vi "Dashboard Main.vi"() -> ()   [LabVIEW 2014]
uses:
  Camera Types.ctl
  <vilib>/event_ctls.llb/eventvkey.ctl
  <vilib>/Rock Robotics/WPI/Dashboard/WPI_DashboardLogging Global.vi
  <vilib>/Rock Robotics/Network Tables/SD Write Number.vi
  <vilib>/Rock Robotics/Network Tables/SD Read Number.vi
  <vilib>/Rock Robotics/Network Tables/SD Write Boolean.vi
  <vilib>/Rock Robotics/Network Tables/SD Read String.vi
  <vilib>/Rock Robotics/Network Tables/SD Write String.vi
  <vilib>/Utility/config.llb/Write Key (String).vi
  <vilib>/Utility/config.llb/Write Key (I32).vi
  <vilib>/Utility/config.llb/NI_LVConfig.lvlib
  <vilib>/vision/NI_Vision_Development_Module.lvlib
panel:
  in  "Limit Tests?":bool
  in  "Camera Type":T1=enum."MS HD3000 square"
  in  "Aspect Fudge Factor":dbl=1.0
  in  "Score Threshold":dbl=75.0
  in  "Show Carpet Mask":bool
  in  "Carpet Color":T2(tab)
  in  "Red":T3={"Hue"={231.0, 14.0}, "Sat"={83.0, 255.0}, "Val"={52.5, 255.0}} {"Hue" scale=0.0..255.0 scale format="%#_3g"}
  in  "Blue":T3={"Hue"={119.0, 181.0}, "Sat"={33.0, 255.0}, "Val"={48.571428571428584, 255.0}} {"Hue" scale=0.0..255.0 scale format="%#_3g"}
  out "Sorted Scores":T4(array[cluster]) {"Carpet" format="%#_3g"; "S" format="%#_3g"; "Trapezoid %" format="%#_3g"; "L" format="%#_3g"; "Area to CH" format="%#_3g"; "X" format="%#_3g"; "Y" format="%#_3g"}
  out "Particles":i32
  out "Masked":T5(plugin-control)
  in  "TCP":refnum<k5>
  in  "Rec Mode":enum32{"Stop", "Record", "Playback"}(radio)
  in  "Vision":u16(ring) items=["Camera Off", "USB Camera SW", "USB Camera HW", "IP Camera"]
  out "Camera IP":string
  out "Image Message":string="Timeout in Camera Communications"
  in  "Dashboard Tab":T6(tab)
  in  "AutonTotePush":bool
  in  "Encoder Reset":bool
  in  "Gyro Reset":bool
  in  "Auton Select":string(combo)="Blank 1"
  out "Drive Mode":string
  in  "Is Logitech":bool
  out "Lift Height":dbl(slide) scale=0.0..4.0
  in  "Camera Settings":T7={"Frame Rate"=30, "Compression"=30, "Size"=1} {"Frame Rate" scale=1.0..30.0; "Size" items=["640x480", "320x240", "160x120"]}
  out "MotorChart R":cluster{"Numeric":dbl, "Numeric":dbl}(graph)
  out "MotorChart L":T8(graph)
  out "MotorSliders R":cluster{"MotorSlide1":dbl, "MotorSlide2":dbl} {"MotorSlide2" scale=-1.0..1.0 scale format="%#_2e"; "MotorSlide1" scale=-1.0..1.0 scale format="%#_2e"}
  out "MotorSliders L":T9 {"MotorSlide4 2" scale=0.0..14.0 scale format="%#_2e"; "MotorSlide2" scale=-1.0..1.0 scale format="%#_2e"; "MotorSlide1" scale=-1.0..1.0 scale format="%#_2e"}
  out "Gyro":dbl(knob) scale=0.0..360.0
  out "JS1 Z":dbl(slide) scale=-1.0..1.0 scale format="%#_2e"
  out "JS1 Graph":cluster{"X":dbl, "Y":dbl}[](graph)
  out "JS1 Buttons":T10
  out "JS2 Z":dbl(slide) scale=-1.0..1.0 scale format="%#_2e"
  out "JS2 Graph":cluster{"X":dbl, "Y":dbl}[](graph)
  out "JS2 Buttons":T10
  out "Mode":T11(ring)=enum."Auto Disabled"
  in  "DB Camera Config":bool
  out "fps":dbl format="%#.1g"
  out "Mbps":dbl format="%#.1g"
  out "Mbps 2":bool
  in  "DB/String 9":string
  in  "DB/String 8":string
  in  "DB/String 7":string
  in  "DB/String 6":string
  in  "DB/String 5":string
  in  "DB/String 4":string
  in  "DB/String 3":string
  in  "DB/String 2":string
  in  "DB/String 1":string
  in  "DB/String 0":string
  in  "DB/Slider 0":dbl(slide) scale=0.0..5.0
  in  "DB/Slider 1":dbl(slide) scale=0.0..5.0
  in  "DB/Slider 2":dbl(slide) scale=0.0..5.0
  in  "DB/Slider 3":dbl(slide) scale=0.0..5.0
  out "DB/LED 3":bool
  out "DB/LED 2":bool
  out "DB/LED 1":bool
  out "DB/LED 0":bool
  in  "DB/Button 3":bool
  in  "DB/Button 2":bool
  in  "DB/Button 1":bool
  in  "DB/Button 0":bool caption="New Name"
  out "Amp Chart":dbl(graph)
  in  "Lift override":bool
  out "Left Lift Current":dbl
  out "Right Lift Current":dbl
  in  "Test Slider":dbl(slide) scale=0.0..100.0 scale format="%#_3g"
  in  "On/Off":bool caption="Solenoid"
  in  "Test Name":u16(ring) items=["Select the test to run...", "Example Test", "-------------------------------", "List of tests is built in robot code.", "Replace with your own automated tests."]
  in  "Test Tree":string(tree)
  in  "Motor":cluster{"Value":dbl, "Enable":bool} {"Value" scale=-1.0..1.0 scale format="%#_3g"}
  out "Progress":T12 {"Test Progress" scale=0.0..100.0}
  in  "Rev/Fwd":cluster{"Forward":bool, "Reverse":bool}
  in  "Test Ring":u16(ring) items=["Monochrome", "Color"]
  in  "Listbox":i32(listbox)
  out "Tree":string(tree)
  in  "Tote Color":T3={"Hue"={23.67058792990901, 48.923317529462665}, "Sat"={66.78571428571429, 255.0}, "Val"={48.571428571428584, 255.0}} {"Hue" scale=0.0..255.0 scale format="%#_3g"}
  in  "Annotate":bool
  out "Detected Totes":T13(array[cluster]) {"Normalized Rect"."Numeric 5" format="%#_2g"; "Normalized Rect"."Numeric 3" format="%#_2g"; "Normalized Rect"."Numeric 2" format="%#_2g"; "Normalized Rect"."Numeric" format="%#_2g"}
  out "Camera Image":T5(plugin-control)
  out "Boolean":bool
  # "Aspect Ratio"
  # "Density Profile"
  # "Left"
  # "Front"
  # "Right"
  # "Battery"
  # "This tab is a great place for autonomous settings and robot-specific values.\nPlace controls and indicators inside this tab and match name to\nDashboard Variables on robot. You can also delete this comment."
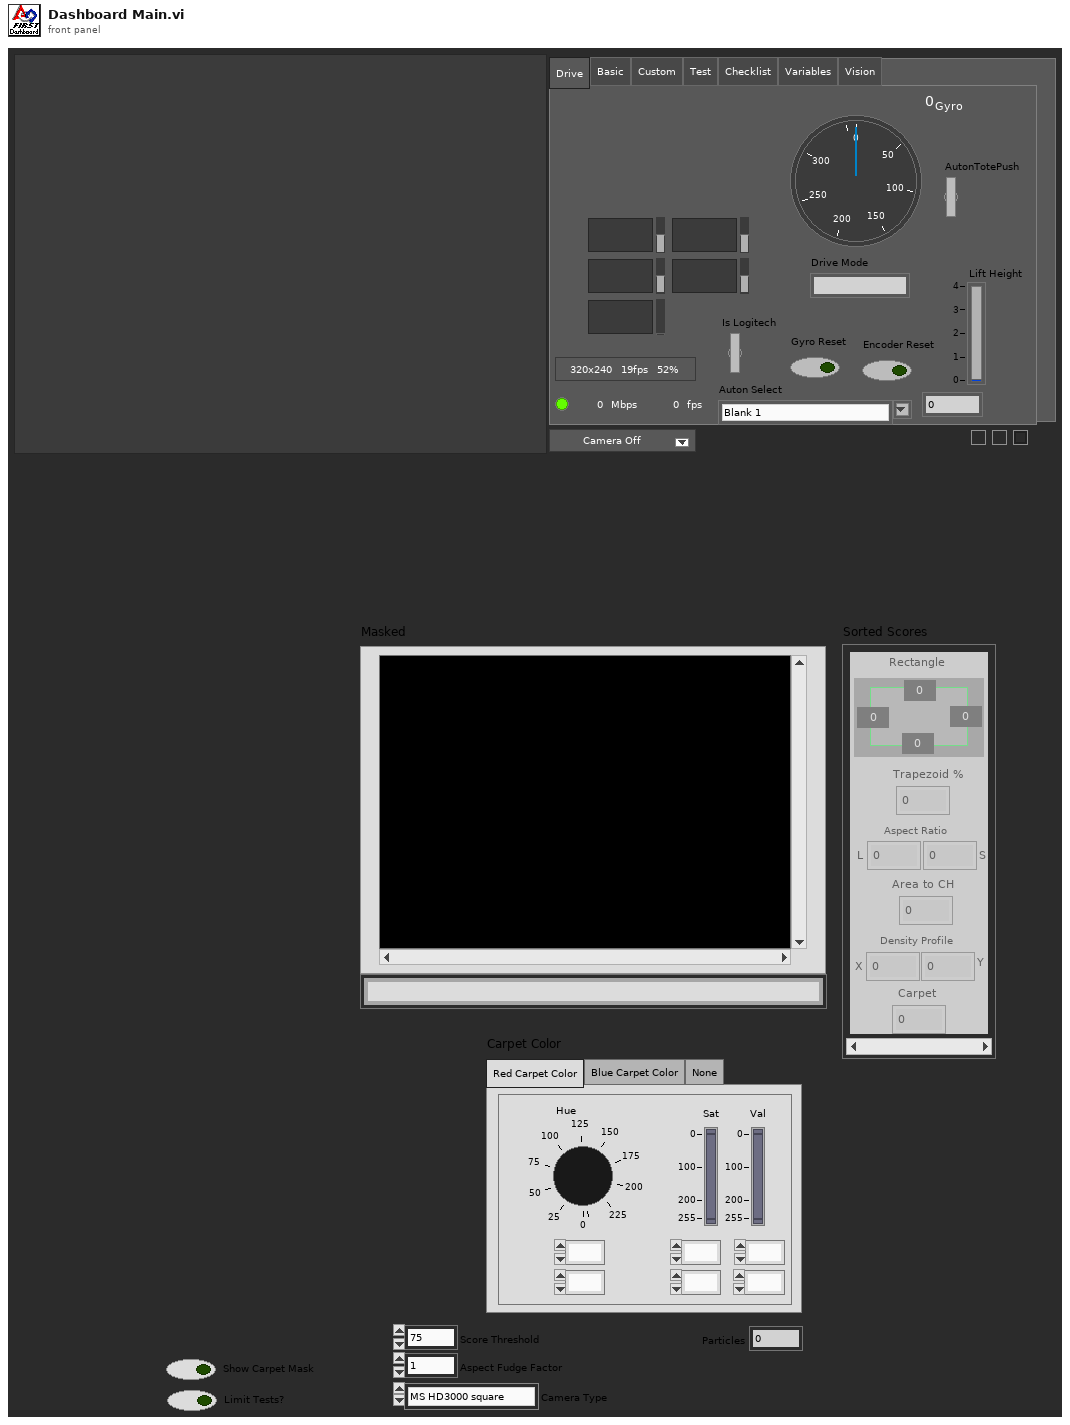
[diagram p1: front panel]
types:
  T1 = typedef "Camera Types.ctl" = enum16{"206", "1011", "1013", "MS HD3000 square", "MS HD3000 640x480"}
  T2 = enum32{"Red Carpet Color", "Blue Carpet Color", "None"}
  T3 = cluster{"Hue":cluster{dbl, dbl}, "Sat":cluster{dbl, dbl}, "Val":cluster{dbl, dbl}}
  T4 = cluster{"Rectangle":cluster{"Numeric":dbl, "Numeric 2":dbl, "Numeric 3":dbl, "Numeric 5":dbl}, "Trapezoid %":dbl, "L":dbl, "S":dbl, "Area to CH":dbl, "X":dbl, "Y":dbl, "Carpet":dbl}[]
  T5 = typedef "IMAQ Image.ctl" = refnum<image>
  T6 = enum32{"Drive", "Basic", "Custom", "Test", "Checklist", "Variables", "Vision"}
  T7 = cluster{"Frame Rate":i32, "Compression":i32, "Size":u16}
  T8 = cluster{"Numeric":dbl, "Numeric":dbl, "Battery V":dbl}
  T9 = cluster{"MotorSlide1":dbl, "MotorSlide2":dbl, "MotorSlide4 2":dbl}
  T10 = cluster{bool, bool, bool, bool, bool, bool, bool, bool, bool, bool, bool, bool}
  T11 = enum8{"Tele-Op Disabled", "Tele-Op Enabled", "Auto Disabled", "Auto Enabled", "Test Disabled", "Test Enabled", "Disconnected", "No Code", "E-Stop"}
  T12 = cluster{"Test Progress":u8, "Test Progress Text":string}
  T13 = cluster{"Distance (ft)":dbl, "Center":cluster{dbl, dbl}, "Normalized Rect":cluster{"Numeric":dbl, "Numeric 2":dbl, "Numeric 3":dbl, "Numeric 5":dbl}}[]
  T14 = typedef "Particle Parameters" = i32
  T15 = typedef "Image Type" = u32
  T16 = enum32{"Drive", "Basic", "Custom", "Test", "Checklist", "Variables"}
  T17 = cluster{"Camera Image":refnum<vi>, "Dashboard Tab":refnum<vi>, "Boolean":refnum<vi>, "Vision":refnum<vi>, "Rec Mode":refnum<vi>, "Test Slider":refnum<vi>, "On/Off ":refnum<vi>, "Test Ring":refnum<vi>, "Rev/Fwd":refnum<vi>, "Test Name":refnum<vi>, "Motor":refnum<vi>, "Progress":refnum<vi>, "CheckList":refnum<vi>, "Tree":refnum<vi>, "Test Tree":refnum<vi>}
  T18 = cluster{"Error Strings":string, "Disable Counts":cluster{u16, u16}, "Rail Faults":cluster{u16, u16, u16}, "Robot IP":string, "DB Mode":u8, "Event Info":cluster{"Name":string, "Type":u8, "Number":u16, "Replay":u8}, "Camera Addr":string}
  T19 = cluster{"Storage":cluster{"Disk Free":u64, "RAM Block":u32, "RAM free":u32}, "CPU Utilization":cluster{"CPU % ISR":sgl, "CPU % Time Crit":sgl, "CPU % Timed Str":sgl, "CPU % High":sgl, "CPU % Above":sgl, "CPU % Normal":sgl, "CPU % Low":sgl}, "CAN":cluster{"% Bus Utilization":sgl, "Bus Off Cnt":u32, "TX_FIFO Full Cnt":u32, "Receive Error Cnt":u8, "Transmit Error Cnt":u8}, "HID":cluster{"HID Outputs":u32, "Rumble Low":u16, "Rumble High":u16}[]}
  T20 = cluster{"Status bits":cluster{"Test Mode":bool, "Autonomous":bool, "Enabled":bool, "Code Start":bool, "Brownout":bool, "Reserved 2":bool, "Reserved 3":bool, "E-Stop":bool}, "Code Trace":cluster{"Disabled":bool, "TeleOp":bool, "Auto":bool, "Test":bool}, "Controller Type":enum16{"unknown", "cRIO", "roboRio"}, "Code?":enum16{"unknown", "noCode", "code"}, "Battery V":dbl}
  T21 = cluster{"Control Bits":cluster{"TestMode":bool, "Autonomous":bool, "Enabled":bool, "FMS Present":bool, bool, bool, bool, "E-Stop":bool}, "Team Station ":u8, "Countdown":sgl, "Joystick Values":cluster{"Axes":dbl[], "Buttons":bool[], "POVs":i16[]}[]}
  T22 = cluster{"Axes":dbl[], "Buttons":bool[], "POVs":i16[]}[]
  T23 = cluster{"Axes":dbl[], "Buttons":bool[], "POVs":i16[]}
  T24 = cluster{"Buttons[0]":bool, "Buttons[1]":bool, "Buttons[2]":bool, "Buttons[3]":bool, "Buttons[4]":bool, "Buttons[5]":bool, "Buttons[6]":bool, "Buttons[7]":bool, "Buttons[8]":bool, "Buttons[9]":bool, "Buttons[10]":bool, "Buttons[11]":bool}
  T25 = cluster{"Bounding box":cluster{"left":dbl, "top":dbl, "right":dbl, "bottom":dbl}, "Trapezoid":dbl, "Long Aspect":dbl, "Short Aspect":dbl, "Area to CH":dbl, "X Mask":dbl, "Y Mask":dbl, "Carpet":dbl}[]
  T26 = cluster{"Red":cluster{"Hue":cluster{dbl, dbl}, "Sat":cluster{dbl, dbl}, "Val":cluster{dbl, dbl}}, "Blue":cluster{"Hue":cluster{dbl, dbl}, "Sat":cluster{dbl, dbl}, "Val":cluster{dbl, dbl}}}
  T27 = cluster{cluster{"[0]":dbl, "[1]":dbl, "[2]":dbl, "[3]":dbl}, "Score":dbl, "Long Edge Score":dbl, "Short Edge Score":dbl, dbl, "X Score":dbl, "Y Score":dbl, "Carpet":dbl}[]
  T28 = cluster{"Distance (ft)":dbl, "Center":cluster{"X":dbl, "Y":dbl}, "Normalized Rect":cluster{"Numeric":dbl, "Numeric 2":dbl, "Numeric 3":dbl, "Numeric 5":dbl}}[]
  T29 = cluster{"Distance (ft)":dbl, "Center":cluster{"X":dbl, "Y":dbl}, "Normalized Rect":cluster{"Numeric":dbl, "Numeric 2":dbl, "Numeric 3":dbl, "Numeric 5":dbl}}
  T30 = typedef "NI_LVConfig.lvlib/Config Data RefNum.ctl" = refnum<k1>
  T31 = cluster{"Operation":enum16{"Update", "Clear"}, "Color Box":u32}[]
  T32 = typedef "eventvkey.ctl" = enum16{"ASCII", "Enter", "Return", "Shift", "Ctrl", "Alt", "Cmd", "Opt", "Caps", "NumLock", "Clear", "Break", "Up", "Down", "Left", "Right", "Insert", "Delete", "Home", "End", "PageUp", "PageDown", "Escape", "Help", "Pause", "ScrollLock", "F1", "F2", "F3", "F4", "F5", "F6", "F7", "F8", "F9", "F10", "F11", "F12", "F13", "F14", "F15", "F16", "F17", "F18", "F19", "F20", "F21", "F22", "F23", "F24", "Play", "VolumeUp", "VolumeDown", "Mute", "Two Byte Char"}
  T33 = cluster{"Image Size":bool, "Image Type":bool, "Pixel Value":bool, "ROI Information":bool, "Zoom Factor":bool}
  T34 = enum8{"Enabled", "Disabled", "Disabled and Grayed Out"}
  T35 = cluster{"Operation":enum16{"Update", "Clear"}, "Color Box":u32}
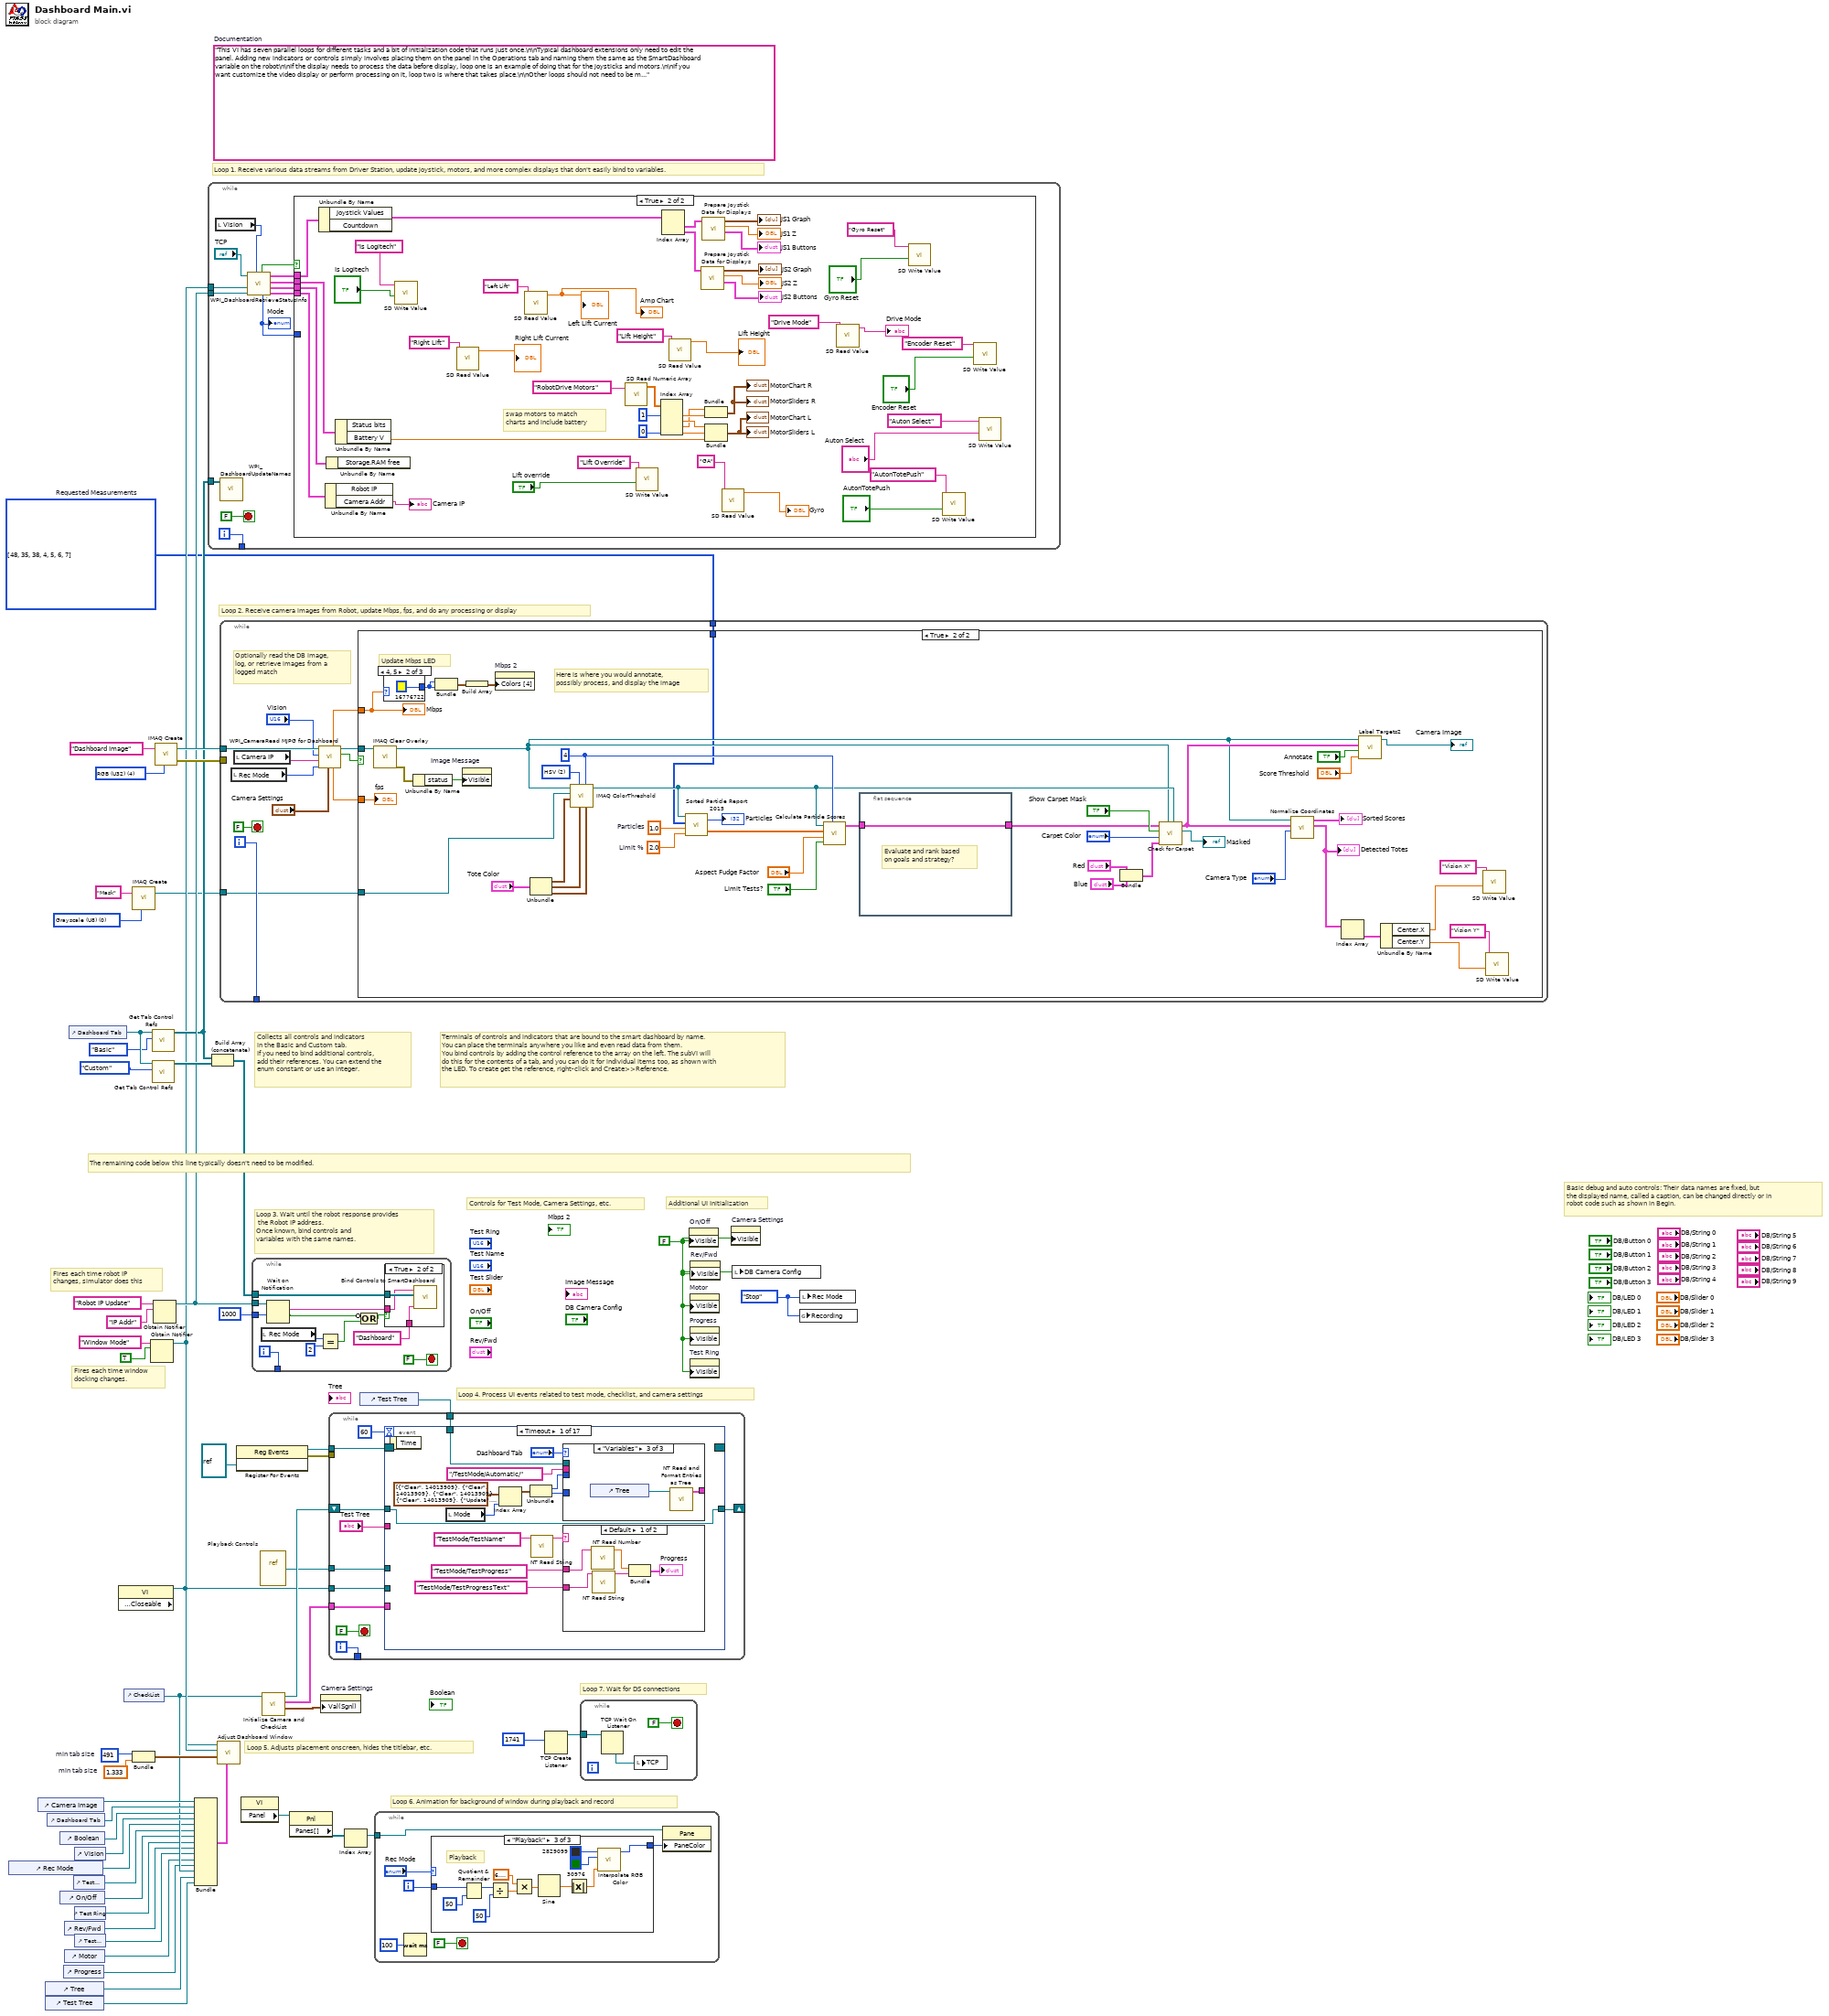
[diagram p0: block diagram]
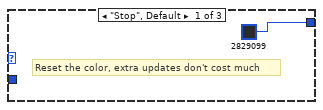
[diagram p3: hidden frame]
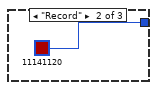
[diagram p4: hidden frame]
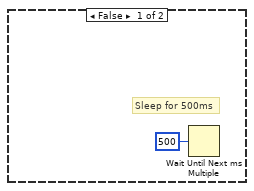
[diagram p6: hidden frame]
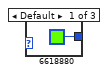
[diagram p7: hidden frame]
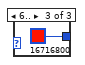
[diagram p8: hidden frame]
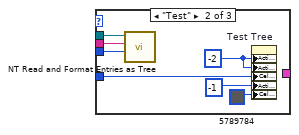
[diagram p10: hidden frame]
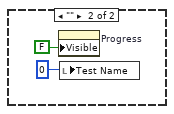
[diagram p11: hidden frame]
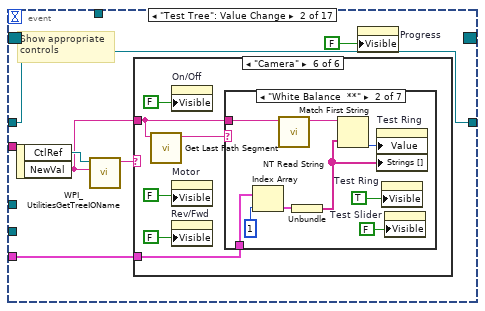
[diagram p12: hidden frame]
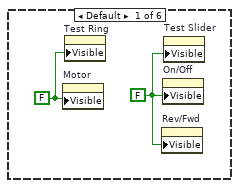
[diagram p13: hidden frame]
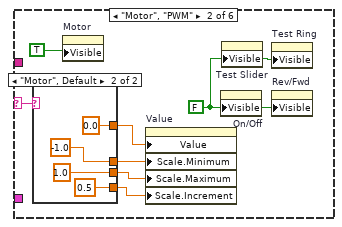
[diagram p14: hidden frame]
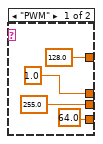
[diagram p15: hidden frame]
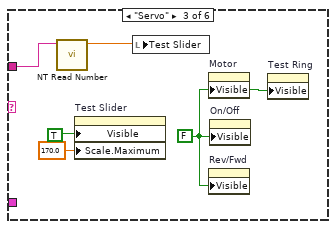
[diagram p16: hidden frame]
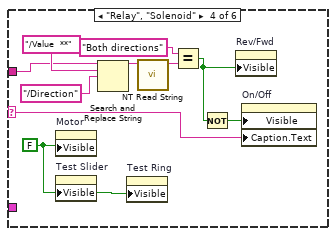
[diagram p17: hidden frame]
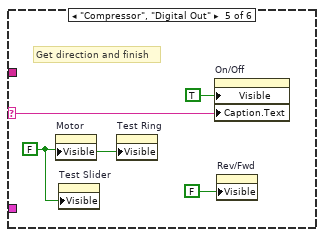
[diagram p18: hidden frame]
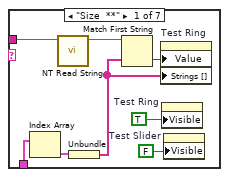
[diagram p19: hidden frame]
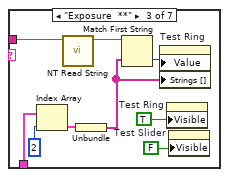
[diagram p20: hidden frame]
diagram:
  w1 = T14[] [48, 35, 38, 4, 5, 6, 7] items=["Center of Mass X", "Center of Mass Y", "First Pixel X", "First Pixel Y", "Bounding Rect Left", "Bounding Rect Top", "Bounding Rect Right", "Bounding Rect Bottom", "Max Feret Diameter Start X", "Max Feret Diameter Start Y", "Max Feret Diameter End X", "Max Feret Diameter End Y", "Max Horiz. Segment Length Left", "Max Horiz. Segment Length Right", "Max Horiz. Segment Length Row", "-", "Bounding Rect Width", "Bounding Rect Height", "Bounding Rect Diagonal", "Perimeter", "Convex Hull Perimeter", "Holes' Perimeter", "Max Feret Diameter", "Equivalent Ellipse Major Axis", "Equivalent Ellipse Minor Axis", "Equivalent Ellipse Minor Axis (Feret)", "Equivalent Rect Long Side", "Equivalent Rect Short Side", "Equivalent Rect Diagonal", "Equivalent Rect Short Side (Feret)", "Average Horiz. Segment Length", "Average Vert. Segment Length", "Hydraulic Radius", "Waddel Disk Diameter", "-", "Area", "Holes' Area", "Particle & Holes' Area", "Convex Hull Area", "Image Area", "-", "Number of Holes", "Number of Horiz. Segments", "Number of Vert. Segments", "-", "Orientation", "Max Feret Diameter Orientation", "-", "% Area/Image Area", "% Area/(Particle & Holes' Area)", "Ratio of Equivalent Ellipse Axes", "Ratio of Equivalent Rect Sides", "-", "Elongation Factor", "Compactness Factor", "Heywood Circularity Factor", "Type Factor", "-", "Sum X", "Sum Y", "Sum XX", "Sum XY", "Sum YY", "Sum XXX", "Sum XXY", "Sum XYY", "Sum YYY", "-", "Moment of Inertia XX", "Moment of Inertia XY", "Moment of Inertia YY", "Moment of Inertia XXX", "Moment of Inertia XXY", "Moment of Inertia XYY", "Moment of Inertia YYY", "Norm. Moment of Inertia XX", "Norm. Moment of Inertia XY", "Norm. Moment of Inertia YY", "Norm. Moment of Inertia XXX", "Norm. Moment of Inertia XXY", "Norm. Moment of Inertia XYY", "Norm. Moment of Inertia YYY", "Hu Moment 1", "Hu Moment 2", "Hu Moment 3", "Hu Moment 4", "Hu Moment 5", "Hu Moment 6", "Hu Moment 7"]  # Requested Measurements
  w4 = T15 0 items=["Grayscale (U8)", "Grayscale (I16)", "Grayscale (SGL)", "Complex (CSG)", "RGB (U32)", "HSL (U32)", "RGB (U64)", "Grayscale (U16)"] ("Image Type")
  w28 = 491  # min tab size
  w27 = 1.333  # min tab size
  w36 = enum32{"Stop", "Record", "Playback"}."Stop" ("Rec Mode")
  w10 = FALSE ("Visible")
  (unwired) "This VI has seven parallel loops for different tasks and a bit of initialization code that runs just once.\n\nTypical dashboard extensions only need to edit the panel. Adding new indicators or controls simply involves placing them on the panel in the Operations tab and naming them the same as the SmartDashboard variable on the robot\n\nIf the display needs to process the data before display, loop one is an example of doing that for the joysticks and motors.\n\nIf you want customize the video display or perform processing on it, loop two is where that takes place.\n\nOther loops should not need to be modified. They are pretty standard, and document the task they perform."  # Documentation
  w56 = T15 4 items=["Grayscale (U8)", "Grayscale (I16)", "Grayscale (SGL)", "Complex (CSG)", "RGB (U32)", "HSL (U32)", "RGB (U64)"] ("Image Type")
  # "Loop 7. Wait for DS connections"
  # "Basic debug and auto controls: Their data names are fixed, but\nthe displayed name, called a caption, can be changed directly or in\nrobot code such as shown in Begin."
  # "Controls for Test Mode, Camera Settings, etc."
  # "Additional UI Initialization"
  # "Loop 6. Animation for background of window during playback and record"
  # "Fires each time robot IP\nchanges, simulator does this"
  # "Fires each time window\ndocking changes."
  # "Collects all controls and indicators\nin the Basic and Custom tab.\nIf you need to bind additional controls,\nadd their references. You can extend the\nenum constant or use an integer."
  # "The remaining code below this line typically doesn't need to be modified."
  # "Loop 4. Process UI events related to test mode, checklist, and camera settings"
  # "Terminals of controls and indicators that are bound to the smart dashboard by name.\nYou can place the terminals anywhere you like and even read data from them.\nYou bind controls by adding the control reference to the array on the left. The subVI will\ndo this for the contents of a tab, and you can do it for individual items too, as shown with\nthe LED. To create get the reference, right-click and Create>>Reference."
  # "Loop 3. Wait until the robot response provides\n the Robot IP address.\nOnce known, bind controls and\nvariables with the same names."
  # "Loop 5. Adjusts placement onscreen, hides the titlebar, etc."
  # "Loop 1. Receive various data streams from Driver Station, update joystick, motors, and more complex displays that don't easily bind to variables."
  # "Loop 2. Receive camera images from Robot, update Mbps, fps, and do any processing or display"
  n1 = control-ref of="Rec Mode"() -> (w16:refnum<vi>)
  n2 = control-ref of="Camera Image"() -> (w31:refnum<vi>)
  n3 = control-ref of="Tree"() -> (w20:refnum<vi>)
  n4 = control-ref of="Test Tree"() -> (w19:refnum<vi>)
  n5 = control-ref of="Dashboard Tab"() -> (w30:refnum<vi>)
  n6 = control-ref of="Boolean"() -> (w25:refnum<vi>)
  n7 = control-ref of="On/Off"() -> (w14:refnum<vi>)
  n8 = control-ref of="Progress"() -> (w11:refnum<vi>)
  n9 = control-ref of="Rev/Fwd"() -> (w12:refnum<vi>)
  n10 = control-ref of="Motor"() -> (w17:refnum<vi>)
  n11 = control-ref of="Dashboard Tab"() -> (w34:refnum<vi>)
  n12 = control-ref of="Test Slider"() -> (w15:refnum<vi>)
  n13 = control-ref of="Vision"() -> (w29:refnum<vi>)
  n14 = control-ref of="Test Ring"() -> (w13:refnum<vi>)
  n15 = control-ref of="Test Name"() -> (w18:refnum<vi>)
  n16 = property class="VI" props=["Front Panel.Closeable"]() -> (reference out=w35:refnum<vi>)  [unwired: 2 in, 2 out]
  n17 = control-ref of="CheckList"() -> (w21:refnum<vi>)
  n18 = call "IMAQ Create"("Image Name"="Mask", "Image Type"=w4) -> ("New Image"=w2:T5)  [unwired: 2 in, 2 out]
  n19 = Bundle("min tab size"=w28, "min tab size"=w27) -> (w26:cluster{"min tab size":i32, "min tab size":dbl})  [unwired: 1 in]
  n20 = Obtain Notifier(name (unnamed)="Window Mode", notification data type=TRUE) -> (notifier out=w7:refnum<notifier>)  [unwired: 2 in, 2 out]
  n21 = call <vilib>:"Get Tab Control Refs.vi"("Page Index"=T16."Basic" ("Dashboard Tab"), "TabControl in"=w34) -> ("ControlsOnPage"=w8:refnum<vi>[])  [unwired: 9 in]
  n22 = call <vilib>:"Get Tab Control Refs.vi"("Page Index"=T16."Custom" ("Dashboard Tab"), "TabControl in"=w34) -> ("ControlsOnPage"=w33:refnum<vi>[])  [unwired: 9 in]
  n23 = Obtain Notifier(name (unnamed)="Robot IP Update", notification data type="IP Addr" ("name (unnamed)")) -> (notifier out=w9:refnum<notifier>)  [unwired: 2 in, 2 out]
  n24 = call "IMAQ Create"("Image Name"="Dashboard Image", "Image Type"=w56) -> ("New Image"=w54:T5, "error out"=w53:errorcluster)  [unwired: 2 in, 1 out]
  n25 = Bundle("Camera Image"=w31, "Dashboard Tab"=w30, "Boolean"=w25, "Vision"=w29, "Rec Mode"=w16, "Test Slider"=w15, "On/Off"=w14, "Test Ring"=w13, "Rev/Fwd"=w12, "Test Name"=w18, "Motor"=w17, "Progress"=w11, "CheckList"=w21, "Tree"=w20, "Test Tree"=w19) -> (w22:T17)  [unwired: 1 in]
  n26 = while {
    tunnel: [w68] -> _
    tunnel: w9 -> [w62]
    tunnel: w8 -> [w61]
    tunnel: w7 -> [w57]
    i -> [w68]
    stop <- FALSE stop-if-true
    n27 = local read "Vision"() -> (w59:u16)
    n28 = call <vilib>:"WPI_DashboardUpdateNames.vi"("Controls on Tab"=w61) -> ()  [unwired: 11 in]
    n29 = call <vilib>:"WPI_DashboardRetrieveStatusInfo.vi"("Vision"=w59, "Binding Refnum"=w62, "Window Mode Notifier"=w57, "TCP Cnx"="TCP") -> ("Power and Errors"=w63:T18, "Robot Metrics"=w66:T19, "Status Info"=w67:T20, "Control Info"=w64:T21, "Robot Mode"=w60:T11, "Process?"=w65:bool)  [unwired: 2 in]
    "Mode" <- w60
    n30 = case shown="True" w65 {
      tunnel: w67 -> [_ w116]
      tunnel: w66 -> [_ w115]
      tunnel: w64 -> [_ w114]
      tunnel: w63 -> [_ w113]
      tunnel: w60 -> [_ _]
      frame False {
      }
      frame True {
        # "swap motors to match\ncharts and include battery"
        n31 = Unbundle By Name(w114) -> ("Joystick Values"=w101:T22)  [unwired: 1 out]
        n32 = Unbundle By Name(w113) -> ("Camera Addr"=→"Camera IP":string)  [unwired: 1 out]
        n33 = Unbundle By Name(w115) -> ()  [unwired: 1 out]
        n34 = Unbundle By Name(w116) -> ("Battery V"=w102:dbl)  [unwired: 1 out]
        n35 = call-poly <vilib>:"SD Write Value.vi"("Boolean"="Is Logitech", "Name"="Is Logitech") -> ()  [unwired: 8 in, 2 out]
        n36 = call-poly <vilib>:"SD Read Value.vi"("Name"="Right Lift") -> ("Numeric"=→"Right Lift Current":dbl)  [unwired: 8 in, 2 out]
        n37 = call-poly <vilib>:"SD Read Value.vi"("Name"="Left Lift") -> ("Numeric"=→"Left Lift Current" →"Amp Chart":dbl)  [unwired: 8 in, 2 out]
        n38 = call <vilib>:"SD Read Numeric Array.vi"("Name"="RobotDrive Motors") -> ("Numeric Array"=w104:dbl[])  [unwired: 8 in, 2 out]
        n39 = call-poly <vilib>:"SD Write Value.vi"("Boolean"="Lift override", "Name"="Lift Override") -> ()  [unwired: 8 in, 2 out]
        n40 = Index Array(array=w104, index #1=1, index #4=0) -> (element #1=w108:dbl, element #2=w109:dbl, element #3=w107:dbl, element #4=w112:dbl)  [unwired: 2 in]
        n41 = Index Array(array=w101) -> (element #1=w100:T23, element #2=w95:T23)  [unwired: 2 in]
        n42 = call-poly <vilib>:"SD Read Value.vi"("Name"="Lift Height") -> ("Numeric"=→"Lift Height":dbl)  [unwired: 8 in, 2 out]
        n43 = call "Prepare Joystick Data for Displays.vi"("Joystick Values"=w95) -> ("Buttons"=→"JS2 Buttons":T24, "Z Axis"=→"JS2 Z":dbl, "Cartesian Data"=→"JS2 Graph":cluster{"X axis":dbl, "X axis":dbl}[])  [unwired: 8 in]
        n44 = call "Prepare Joystick Data for Displays.vi"("Joystick Values"=w100) -> ("Buttons"=→"JS1 Buttons":T24, "Z Axis"=→"JS1 Z":dbl, "Cartesian Data"=→"JS1 Graph":cluster{"X axis":dbl, "X axis":dbl}[])  [unwired: 8 in]
        n45 = Bundle("Numeric"=w107, "Numeric"=w108) -> (→"MotorChart R" →"MotorSliders R":cluster{"Numeric":dbl, "Numeric":dbl})  [unwired: 1 in]
        n46 = Bundle("Numeric"=w109, "Numeric"=w112, "Battery V"=w102) -> (→"MotorChart L" →"MotorSliders L":T8)  [unwired: 1 in]
        n47 = call-poly <vilib>:"SD Read Value.vi"("Name"="GA") -> ("Numeric"=→"Gyro":dbl)  [unwired: 8 in, 2 out]
        n48 = call-poly <vilib>:"SD Read Value.vi"("Name"="Drive Mode") -> ("String"=→"Drive Mode":string)  [unwired: 8 in, 2 out]
        n49 = call-poly <vilib>:"SD Write Value.vi"("Boolean"="Gyro Reset", "Name"="Gyro Reset") -> ()  [unwired: 8 in, 2 out]
        n50 = call-poly <vilib>:"SD Write Value.vi"("Boolean"="AutonTotePush", "Name"="AutonTotePush") -> ()  [unwired: 8 in, 2 out]
        n51 = call-poly <vilib>:"SD Write Value.vi"("Boolean"="Encoder Reset", "Name"="Encoder Reset" ("Table Prefix")) -> ()  [unwired: 8 in, 2 out]
        n52 = call-poly <vilib>:"SD Write Value.vi"("String"="Auton Select", "Name"="Auton Select") -> ()  [unwired: 8 in, 2 out]
      }
    }
  }
  n53 = Build Array (concatenate)(w8, w33) -> (w32:refnum<vi>[])
  n54 = call "Adjust Dashboard Window.vi"("Sizing Refnums"=w22, "Size Constraints"=w26, "VI"=w35, "Notifier in"=w7) -> ()  [unwired: 8 in]
  n55 = while {
    tunnel: w54 -> [w127]
    tunnel: w53 -> [_]
    tunnel: [w128] -> _
    tunnel: w2 -> [w118]
    tunnel: w1 -> [w117]
    i -> [w128]
    stop <- FALSE stop-if-true
    # "Optionally read the DB image,\nlog, or retrieve images from a\nlogged match"
    n56 = local read "Rec Mode"() -> (w121:enum32{"Stop", "Record", "Playback"})
    n57 = local read "Camera IP"() -> (w119:string)
    n58 = call <vilib>:"WPI_CameraRead MJPG for Dashboard.vi"("Camera Settings"="Camera Settings", "Rec Mode"=w121, "Camera IP"=w119, "Camera Mode"="Vision", "Refnum in"=w127) -> ("Active"=w125:bool, "Refnum out"=w126:T5, "FPS"=w124:dbl, "Bandwidth (Mbps)"=w123:dbl)  [unwired: 3 in]
    n59 = case shown="True" w125 {
      tunnel: w126 -> [_ w169]
      tunnel: w123 -> [_ w168]
      tunnel: w124 -> [_ w167]
      tunnel: w118 -> [_ w139]
      tunnel: w117 -> [_ w137]
      frame False {
        # "Sleep for 500ms"
        n60 = Wait Until Next ms Multiple(millisecond multiple=u32 500) -> ()  [unwired: 1 out]
      }
      frame True {
        w152 = 4 ("Replace Value")
        w159 = 2.0  # Limit %
        w162 = 1.0  # Particles
        w166 = u16 2 items=["RGB", "HSL", "HSV", "HSI"] ("Color Mode")
        # "Here is where you would annotate,\npossibly process, and display the image"
        # "Update Mbps LED"
        n61 = call "IMAQ Clear Overlay"("Image"=w169) -> ("error out"=w173:errorcluster, "Image Out"=w141:T5)  [unwired: 2 in, 7 out]
        n62 = case shown="4, 5" w168 {
          tunnel: [u32 6618880 ("Color Box") u32 16776722 ("Color Box") u32 16716800 ("Color Box")] -> w170
          frame Default {
          }
          frame 4, 5 {
          }
          frame 6.. {
          }
        }
        n63 = Unbundle By Name(w173) -> ("status"=w174:bool)
        n64 = Bundle("Color Box"=w170, "Color Box"=w170) -> (w172:cluster{"Color Box":u32, "Color Box":u32})  [unwired: 1 out]
        n65 = property on="Image Message" class="Str"("Visible"=w174) -> ()  [unwired: 2 in, 2 out]
        n66 = Build Array(w172) -> (w171:cluster{"Color Box":u32, "Color Box":u32}[])
        n67 = property on="Mbps 2" class="Bool (strict)"("Colors [4]"=w171) -> ()  [unwired: 2 in, 2 out]
        n68 = Unbundle("Tote Color") -> ("Hue"=w165:cluster{dbl, dbl}, "Sat"=w164:cluster{dbl, dbl}, "Val"=w163:cluster{dbl, dbl})
        n69 = call "IMAQ ColorThreshold"("Blue or Luma or Val or Inten Range"=w163, "Replace Value"=w152, "Green or Sat Range"=w164, "Color Mode"=w166, "Red or Hue Range"=w165, "Image Dst"=w139, "Image Src"=w141) -> ("Image Dst Out"=w145:T5)  [unwired: 3 in, 1 out]
        n70 = call "Sorted Particle Report 2015.vi"("Min Area Size %"=w159, "Particle Count Limit"=w162, "Pixel Measurements"=w137, "Image in"=w145) -> ("Sorted Data"=w160:dbl[][], "Particles"=→"Particles":i32)
        n71 = call "Calculate Particle Scores.vi"("Pixel Value"=w152, "Limit Tests?"="Limit Tests?", "Aspect Fudge Factor"="Aspect Fudge Factor", "Sorted Data"=w160, "Image in"=w145) -> ("Scores"=w147:T25)  [unwired: 6 in]
        n72 = flat-sequence {
          tunnel: w147 -> [w175]
          tunnel: [w175] -> w146
          frame #0 {
            # "Evaluate and rank based\non goals and strategy?"
          }
        }
        n73 = Bundle("Red"="Red", "Blue"="Blue") -> (w153:T26)  [unwired: 1 in]
        n74 = call "Check for Carpet.vi"("Original Mask"=w145, "Original Color"=w141, "Carpet Colors"=w153, "Carpet Selector"="Carpet Color", "Combine Carpet Mask"="Show Carpet Mask", "Initial Scores"=w146) -> ("Updated Mask"=→"Masked":T5, "Updated Scores"=w151:T27)  [unwired: 4 in]
        n75 = call "Normalize Coordinates.vi"("Camera Type"="Camera Type", "Targets"=w151, "Image in"=w141) -> ("Found Totes"=w135:T28, "Sorted Scores"=→"Sorted Scores":T4)  [unwired: 7 in]
        "Detected Totes" <- w135
        n76 = Index Array(array=w135) -> (element=w138:T29)  [unwired: 1 in]
        n77 = call "Label Targets2.vi"("Score Threshold"="Score Threshold", "Annotate"="Annotate", "Targets"=w151, "Image in"=w141) -> ("Image out"=→"Camera Image":T5)  [unwired: 7 in]
        n78 = Unbundle By Name(w138) -> ("Center.X"=w133:dbl, "Center.Y"=w134:dbl)
        n79 = call-poly <vilib>:"SD Write Value.vi"("Numeric"=w133, "Name"="Vision X") -> ()  [unwired: 8 in, 2 out]
        n80 = call-poly <vilib>:"SD Write Value.vi"("Numeric"=w134, "Name"="Vision Y") -> ()  [unwired: 8 in, 2 out]
        "Mbps" <- w168
        "fps" <- w167
      }
    }
  }
  n81 = register-events(refnum<vi> refnum) -> (reference out=w40:refnum<event-registration>, error out=w39:errorcluster)  [unwired: 2 in]
  n82 = property class="VI"() -> ("Panel"=w43:refnum<vi>)  [unwired: 2 in, 2 out]
  n83 = while {
    tunnel: w32 -> [w190]
    tunnel: w9 -> [w188]
    tunnel: [w186] -> _
    tunnel: u32 1000 ("milliseconds to wait") -> [w185]
    i -> [w186]
    stop <- FALSE stop-if-true
    n84 = local read "Rec Mode"() -> (w181:enum32{"Stop", "Record", "Playback"})
    n85 = Wait on Notification(notifier=w188, timeout in ms (-1)=w185) -> (notification=w187:string, timed out?=w183:bool)  [unwired: 2 in, 2 out]
    n86 = Equal?(x=w181, y=u16 2 ("Rec Mode")) -> (x = y?=w182:bool)
    n87 = Compound Arithmetic op=OR(invert w183, w182) -> (w184:bool)
    n88 = case shown="True" w184 {
      tunnel: w190 -> [_ w193]
      tunnel: w187 -> [_ w192]
      tunnel: "Dashboard" -> [_ w191]
      frame False {
      }
      frame True {
        n89 = call <vilib>:"Bind Controls to SmartDashboard.vi"("Client Name"=w191, "Bound Control Refs"=w193, "Server IP Address"=w192) -> ()  [unwired: 9 in]
      }
    }
  }
  n90 = vi-ref "Playback Controls.vi"() -> (w41:refnum<vi>)
  n91 = call "Initialize Camera and CheckList.vi"("ListBox in"=w21) -> ("Cluster"=w47:cluster{"value":i32, "value":i32, "index":i32}, "Array"=w48:cluster{string[]}[], "File Refnum"=w46:T30)  [unwired: 8 in]
  n92 = property class="Pnl"(reference=w43) -> ("Panes[]"=w44:refnum<vi>[])  [unwired: 1 in, 2 out]
  n93 = property on="Camera Settings" class="Clust (strict)"("Val(Sgnl)"=w47) -> ()  [unwired: 2 in, 2 out]
  n94 = Index Array(array=w44) -> (element=w42:refnum<vi>)  [unwired: 1 in]
  n95 = control-ref of="Test Tree"() -> (w45:refnum<vi>)
  n96 = while {
    tunnel: w48 -> [w201]
    shift-right: [w200] -> _
    shift-left: w46 -> [w199]
    tunnel: [w198] -> _
    tunnel: w45 -> [w197]
    tunnel: w41 -> [w196]
    tunnel: w40 -> [w195]
    tunnel: w39 -> [_]
    tunnel: w35 -> [w194]
    i -> [w198]
    stop <- FALSE stop-if-true
    n97 = event shown="[0] Timeout" {
      selector: w195 -> [_ _ _ _ _ _ _ _ _ _ _ _ _ _ _ _ _]
      dyn-events: [_ _ _ _ _ _ _ _ _ _ _ _ _ w439 _ _ _] -> _
      timeout: u32 60 ("milliseconds to wait") -> [_ _ _ _ _ _ _ _ _ _ _ _ _ _ _ _ _]
      tunnel: w197 -> [w213 _ _ _ _ _ _ _ _ _ _ _ _ _ _ _ _]
      tunnel: "Test Tree" -> [_ _ _ _ _ _ _ _ w408 w416 w418 w422 w430 _ _ _ _]
      tunnel: w201 -> [_ w235 _ _ _ _ w372 w402 _ _ _ _ _ _ _ _ _]
      tunnel: [w209 w234 w333 w338 w346 w358 w371 w395 w407 w414 w417 w421 w429 w441 w455 w456 w466] -> w200
      tunnel: w199 -> [w209 w234 w333 w338 w346 w358 w370 w395 w407 w414 w417 w421 w429 w441 w455 w456 w466]
      tunnel: w196 -> [_ _ _ _ _ _ _ _ _ _ _ _ _ w442 _ w459 _]
      tunnel: w194 -> [_ _ _ _ _ _ _ _ _ _ _ _ _ w437 _ _ _]
      event Timeout {
        n98 = event-data() -> ()  [unwired: 1 in, 1 out]
        n99 = local read "Mode"() -> (w212:T11)
        n100 = Index Array(array=T31 [{"Operation"=enum."Clear", "Color Box"=14013909}, {"Operation"=enum."Clear", "Color Box"=14013909}, {"Operation"=enum."Clear", "Color Box"=14013909}, {"Operation"=enum."Clear", "Color Box"=14013909}, {"Operation"=enum."Update", "Color Box"=14013909}, {"Operation"=enum."Update", "Color Box"=16777215}, {"Operation"=enum."Clear", "Color Box"=14013909}, {"Operation"=enum."Clear", "Color Box"=14013909}, {"Operation"=enum."Clear", "Color Box"=14013909}], index=w212) -> (element=w207:T35)
        n101 = Unbundle(w207) -> ("Operation"=w206:enum16{"Update", "Clear"}, "Color Box"=w205:u32)
        n102 = call <vilib>:"NT Read String.vi"("Name"="TestMode/TestName") -> ("String"=w216:string)  [unwired: 9 in, 1 out]
        n103 = case shown="\"Variables\"" "Dashboard Tab" {
          tunnel: w213 -> [_ w224 _]
          tunnel: "/TestMode/Automatic/" ("Name Pattern") -> [_ w223 _]
          tunnel: w206 -> [_ w222 _]
          tunnel: [_ _ w226] -> _
          tunnel: w205 -> [_ w218 _]
          frame "Custom", Default {
          }
          frame "Test" {
            w221 = -2 ("Active Item:Row Number")
            n104 = call <vilib>:"NT Read and Format Entries as Tree.vi"("Operation"=w222, "Name Pattern"=w223, "Tree Refnum"=w224) -> ()  [unwired: 7 in, 2 out]
            n105 = property on="Test Tree" class="Tree (strict)"("Active Item Row Number"=w221, "ActiveColNum"=w221, "CellBG"=w218, "Active Item Row Number"=-1 ("Active Item:Row Number"), "CellBG"=u32 5789784 ("Color Box")) -> ()  [unwired: 2 in, 2 out]
          }
          frame "Variables" {
            n106 = control-ref of="Tree"() -> (w225:refnum<vi>)
            n107 = call <vilib>:"NT Read and Format Entries as Tree.vi"("Tree Refnum"=w225) -> ("Formatted Strings"=w226:cluster{"Name":string, "Value":string}[])  [unwired: 9 in, 1 out]
          }
        }
        n108 = case shown="Default" w216 {
          tunnel: "TestMode/TestProgress" ("Name") -> [w228 _]
          tunnel: "TestMode/TestProgressText" ("Name") -> [w227 _]
          frame Default {
            n109 = call <vilib>:"NT Read Number.vi"("Name"=w228) -> ("Numeric"=w229:dbl)  [unwired: 9 in, 1 out]
            n110 = call <vilib>:"NT Read String.vi"("Name"=w227) -> ("String"=w230:string)  [unwired: 9 in, 1 out]
            n111 = Bundle("Numeric"=w229, "String"=w230) -> (→"Progress":cluster{"Numeric":dbl, "String":string})  [unwired: 1 in]
          }
          frame "" {
            n112 = property on="Progress" class="Clust (strict)"("Visible"=FALSE) -> ()  [unwired: 2 in, 2 out]
            n113 = local write "Test Name"(u16 0) -> ()
          }
        }
      }
      event "Test Tree": Value Change {
        # "Show appropriate\ncontrols"
        n114 = event-data() -> ("CtlRef"=w238:refnum<vi>, "NewVal"=w236:string)  [unwired: 1 in]
        n115 = call <vilib>:"WPI_UtilitiesGetTreeIOName.vi"("NewVal"=w236, "TreeControl in"=w238) -> ("I/O Name"=w239:string)  [unwired: 9 in]
        n116 = case shown="\"Camera\"" w239 {
          selector: w239 -> [_ w246 _ w264 w273 _]
          tunnel: w236 -> [_ _ w261 w263 _ w280]
          tunnel: w235 -> [_ _ _ _ _ w279]
          frame Default {
            w241 = FALSE ("Visible")
            w240 = FALSE ("Visible")
            n117 = property on="Motor" class="Clust (strict)"("Visible"=w240) -> ()  [unwired: 2 in, 2 out]
            n118 = property on="Test Ring" class="Ring (strict)"("Visible"=w240) -> ()  [unwired: 2 in, 2 out]
            n119 = property on="Rev/Fwd" class="Clust (strict)"("Visible"=w241) -> ()  [unwired: 2 in, 2 out]
            n120 = property on="On/Off" class="Bool (strict)"("Visible"=w241) -> ()  [unwired: 2 in, 2 out]
            n121 = property on="Test Slider" class="Slide (strict)"("Visible"=w241) -> ()  [unwired: 2 in, 2 out]
          }
          frame "Motor", "PWM" {
            w247 = FALSE ("Visible")
            n122 = case shown="\"Motor\", Default" w246 {
              tunnel: [1.0 ("Value") -1.0 ("Value")] -> w245
              tunnel: [255.0 ("Value") 1.0 ("Value")] -> w244
              tunnel: [128.0 ("Value") 0.0 ("Value")] -> w243
              tunnel: [64.0 ("Value") 0.5 ("Value")] -> w242
              frame "PWM" {
              }
              frame "Motor", Default {
              }
            }
            n123 = property on="Motor" class="Clust (strict)"("Visible"=TRUE) -> ()  [unwired: 2 in, 2 out]
            n124 = property on="Value" class="Slide (strict)"("Value"=w243, "Scale.Minimum"=w245, "Scale.Maximum"=w244, "Scale.Increment"=w242) -> ()  [unwired: 2 in, 2 out]
            n125 = property on="On/Off" class="Bool (strict)"("Visible"=w247) -> ()  [unwired: 2 in, 2 out]
            n126 = property on="Test Slider" class="Slide (strict)"("Visible"=w247) -> ()  [unwired: 2 in, 2 out]
            n127 = property on="Test Ring" class="Ring (strict)"("Visible"=w247) -> ()  [unwired: 2 in, 2 out]
            n128 = property on="Rev/Fwd" class="Clust (strict)"("Visible"=w247) -> ()  [unwired: 2 in, 2 out]
          }
          frame "Servo" {
            w259 = FALSE ("Visible")
            n129 = call <vilib>:"NT Read Number.vi"("Name"=w261) -> ("Numeric"=w260:dbl)  [unwired: 9 in, 1 out]
            n130 = property on="Test Slider" class="Slide (strict)"("Visible"=TRUE, "Scale.Maximum"=170.0 ("Scale.Range:Maximum")) -> ()  [unwired: 2 in, 2 out]
            n131 = local write "Test Slider"(w260) -> ()
            n132 = property on="Motor" class="Clust (strict)"("Visible"=w259) -> ()  [unwired: 2 in, 2 out]
            n133 = property on="Rev/Fwd" class="Clust (strict)"("Visible"=w259) -> ()  [unwired: 2 in, 2 out]
            n134 = property on="On/Off" class="Bool (strict)"("Visible"=w259) -> ()  [unwired: 2 in, 2 out]
            n135 = property on="Test Ring" class="Ring (strict)"("Visible"=w259) -> ()  [unwired: 2 in, 2 out]
          }
          frame "Relay", "Solenoid" {
            w262 = FALSE ("Visible")
            n136 = property on="Motor" class="Clust (strict)"("Visible"=w262) -> ()  [unwired: 2 in, 2 out]
            n137 = property on="Test Slider" class="Slide (strict)"("Visible"=w262) -> ()  [unwired: 2 in, 2 out]
            n138 = Search and Replace String(input string=w263, search string="/Value  **", replace string="/Direction") -> (result string=w269:string)  [unwired: 5 in, 3 out]
            n139 = property on="Test Ring" class="Ring (strict)"("Visible"=w262) -> ()  [unwired: 2 in, 2 out]
            n140 = call <vilib>:"NT Read String.vi"("Name"=w269) -> ("String"=w267:string)  [unwired: 9 in, 1 out]
            n141 = Equal?(x="Both directions", y=w267) -> (x = y?=w265:bool)
            n142 = Not(x=w265) -> (.not. x?=w266:bool)
            n143 = property on="Rev/Fwd" class="Clust (strict)"("Visible"=w265) -> ()  [unwired: 2 in, 2 out]
            n144 = property on="On/Off" class="Bool (strict)"("Visible"=w266, "Caption.Text"=w264) -> ()  [unwired: 2 in, 2 out]
          }
          frame "Compressor", "Digital Out" {
            w272 = FALSE ("Visible")
            # "Get direction and finish"
            n145 = property on="Motor" class="Clust (strict)"("Visible"=w272) -> ()  [unwired: 2 in, 2 out]
            n146 = property on="Test Slider" class="Slide (strict)"("Visible"=w272) -> ()  [unwired: 2 in, 2 out]
            n147 = property on="Test Ring" class="Ring (strict)"("Visible"=w272) -> ()  [unwired: 2 in, 2 out]
            n148 = property on="On/Off" class="Bool (strict)"("Visible"=TRUE, "Caption.Text"=w273) -> ()  [unwired: 2 in, 2 out]
            n149 = property on="Rev/Fwd" class="Clust (strict)"("Visible"=FALSE) -> ()  [unwired: 2 in, 2 out]
          }
          frame "Camera" {
            n150 = call <vilib>:"Get Last Path Segment.vi"("String in"=w280) -> ("String out"=w281:string)  [unwired: 10 in]
            n151 = property on="On/Off" class="Bool (strict)"("Visible"=FALSE) -> ()  [unwired: 2 in, 2 out]
            n152 = property on="Motor" class="Clust (strict)"("Visible"=FALSE) -> ()  [unwired: 2 in, 2 out]
            n153 = property on="Rev/Fwd" class="Clust (strict)"("Visible"=FALSE) -> ()  [unwired: 2 in, 2 out]
            n154 = case shown="\"White Balance  **\"" w281 {
              tunnel: w280 -> [w287 w296 w305 w314 w323 _ w329]
              tunnel: w279 -> [w285 w293 w302 w311 w320 _ _]
              frame "Size  **" {
                n155 = Index Array(array=w285) -> (element=w284:cluster{string[]})  [unwired: 1 in]
                n156 = call <vilib>:"NT Read String.vi"("Name"=w287) -> ("String"=w286:string)  [unwired: 9 in, 1 out]
                n157 = Unbundle(w284) -> (w282:string[])
                n158 = Match First String(2:w282, 3:w286) -> (0:w283:i32)  [unwired: 1 out]
                n159 = property on="Test Ring" class="Ring (strict)"("Value"=w283, "Strings []"=w282) -> ()  [unwired: 2 in, 2 out]
                n160 = property on="Test Ring" class="Ring (strict)"("Visible"=TRUE) -> ()  [unwired: 2 in, 2 out]
                n161 = property on="Test Slider" class="Slide (strict)"("Visible"=FALSE) -> ()  [unwired: 2 in, 2 out]
              }
              frame "White Balance  **" {
                n162 = Index Array(array=w293, index=1) -> (element=w294:cluster{string[]})
                n163 = call <vilib>:"NT Read String.vi"("Name"=w296) -> ("String"=w295:string)  [unwired: 9 in, 1 out]
                n164 = Unbundle(w294) -> (w291:string[])
                n165 = Match First String(2:w291, 3:w295) -> (0:w290:i32)  [unwired: 1 out]
                n166 = property on="Test Ring" class="Ring (strict)"("Value"=w290, "Strings []"=w291) -> ()  [unwired: 2 in, 2 out]
                n167 = property on="Test Ring" class="Ring (strict)"("Visible"=TRUE) -> ()  [unwired: 2 in, 2 out]
                n168 = property on="Test Slider" class="Slide (strict)"("Visible"=FALSE) -> ()  [unwired: 2 in, 2 out]
              }
              frame "Exposure  **" {
                n169 = Index Array(array=w302, index=2) -> (element=w303:cluster{string[]})
                n170 = call <vilib>:"NT Read String.vi"("Name"=w305) -> ("String"=w304:string)  [unwired: 9 in, 1 out]
                n171 = Unbundle(w303) -> (w299:string[])
                n172 = Match First String(2:w299, 3:w304) -> (0:w300:i32)  [unwired: 1 out]
                n173 = property on="Test Ring" class="Ring (strict)"("Value"=w300, "Strings []"=w299) -> ()  [unwired: 2 in, 2 out]
                n174 = property on="Test Ring" class="Ring (strict)"("Visible"=TRUE) -> ()  [unwired: 2 in, 2 out]
                n175 = property on="Test Slider" class="Slide (strict)"("Visible"=FALSE) -> ()  [unwired: 2 in, 2 out]
              }
              frame "Exposure Priority  **" {
                n176 = Index Array(array=w311, index=3) -> (element=w312:cluster{string[]})
                n177 = call <vilib>:"NT Read String.vi"("Name"=w314) -> ("String"=w313:string)  [unwired: 9 in, 1 out]
                n178 = Unbundle(w312) -> (w308:string[])
                n179 = Match First String(2:w308, 3:w313) -> (0:w309:i32)  [unwired: 1 out]
                n180 = property on="Test Ring" class="Ring (strict)"("Value"=w309, "Strings []"=w308) -> ()  [unwired: 2 in, 2 out]
                n181 = property on="Test Ring" class="Ring (strict)"("Visible"=TRUE) -> ()  [unwired: 2 in, 2 out]
                n182 = property on="Test Slider" class="Slide (strict)"("Visible"=FALSE) -> ()  [unwired: 2 in, 2 out]
              }
              frame "Color Enable  **" {
                n183 = Index Array(array=w320, index=4) -> (element=w321:cluster{string[]})
                n184 = call <vilib>:"NT Read String.vi"("Name"=w323) -> ("String"=w322:string)  [unwired: 9 in, 1 out]
                n185 = Unbundle(w321) -> (w317:string[])
                n186 = Match First String(2:w317, 3:w322) -> (0:w318:i32)  [unwired: 1 out]
                n187 = property on="Test Ring" class="Ring (strict)"("Value"=w318, "Strings []"=w317) -> ()  [unwired: 2 in, 2 out]
                n188 = property on="Test Ring" class="Ring (strict)"("Visible"=TRUE) -> ()  [unwired: 2 in, 2 out]
                n189 = property on="Test Slider" class="Slide (strict)"("Visible"=FALSE) -> ()  [unwired: 2 in, 2 out]
              }
              frame Default {
                n190 = property on="Test Ring" class="Ring (strict)"("Visible"=FALSE) -> ()  [unwired: 2 in, 2 out]
                n191 = property on="Test Slider" class="Slide (strict)"("Visible"=FALSE) -> ()  [unwired: 2 in, 2 out]
              }
              frame "Brightness  **", "Color Level  **", "Compression  **", "FPS  **", "Sharpness  **" {
                n192 = call <vilib>:"NT Read Number.vi"("Name"=w329) -> ("Numeric"=w328:dbl)  [unwired: 9 in, 1 out]
                n193 = local write "Test Slider"(w328) -> ()
                n194 = property on="Test Slider" class="Slide (strict)"("Visible"=TRUE, "Scale.Maximum"=100.0 ("Scale.Range:Maximum")) -> ()  [unwired: 2 in, 2 out]
                n195 = property on="Test Ring" class="Ring (strict)"("Visible"=FALSE) -> ()  [unwired: 2 in, 2 out]
              }
            }
          }
        }
        n196 = property on="Progress" class="Clust (strict)"("Visible"=FALSE) -> ()  [unwired: 2 in, 2 out]
      }
      event "Test Name": Mouse Enter {
        # "Populate the ring with the list of tests"
        n197 = event-data() -> ()  [unwired: 1 in, 1 out]
        n198 = call <vilib>:"NT Read String Array.vi"("Name"="TestMode/TestList") -> ("String Array"=w337:string[])  [unwired: 9 in, 1 out]
        n199 = Build Array (concatenate)("Select the test to run...", w337) -> (w336:string[])
        n200 = property on="Test Name" class="Ring (strict)"("Strings []"=w336) -> ()  [unwired: 2 in, 2 out]
      }
      event "Test Name": Value Change {
        w339 = FALSE ("Visible")
        # "Tell the robot the test name to run"
        n201 = event-data() -> ("NewVal"=w343:u16)  [unwired: 1 in]
        n202 = property on="Test Name" class="Ring (strict)"() -> ("Strings []"=w344:string[])  [unwired: 2 in, 2 out]
        n203 = local write "Progress"(T12 {"Test Progress"=0, "Test Progress Text"=""} ("Progress")) -> ()
        n204 = Index Array(array=w344, index=w343) -> (element=w342:string)
        n205 = call <vilib>:"NT Write String.vi"("String"=w342, "Name"="TestMode/TestName") -> ()  [unwired: 9 in, 1 out]
        n206 = property on="Progress" class="Clust (strict)"("Visible"=TRUE) -> ()  [unwired: 2 in, 2 out]
        n207 = property on="Motor" class="Clust (strict)"("Visible"=w339) -> ()  [unwired: 2 in, 2 out]
        n208 = property on="Test Slider" class="Slide (strict)"("Visible"=w339) -> ()  [unwired: 2 in, 2 out]
        n209 = property on="On/Off" class="Bool (strict)"("Visible"=w339) -> ()  [unwired: 2 in, 2 out]
        n210 = property on="Rev/Fwd" class="Clust (strict)"("Visible"=w339) -> ()  [unwired: 2 in, 2 out]
        n211 = property on="Test Ring" class="Ring (strict)"("Visible"=w339) -> ()  [unwired: 2 in, 2 out]
      }
      event "Listbox": Double Click {
        # "Shift clears all"
        # "Update symbols on the listbox"
        n212 = event-data() -> ("PlatMods.Shift"=w347:bool, "Row"=w349:i32)  [unwired: 1 in]
        n213 = case shown="True" w347 {
          tunnel: w349 -> [w353 _]
          tunnel: 1 -> [w352 _]
          frame False {
            n214 = property on="Listbox" class="LstBox (strict)"() -> ("Item Symbols"=w351:i32[])  [unwired: 2 in, 2 out]
            n215 = Replace Array Subset(array=w351, new element=w352, index=w353) -> (w350:i32[])
            n216 = property on="Listbox" class="LstBox (strict)"("Item Symbols"=w350) -> ()  [unwired: 2 in, 2 out]
          }
          frame True {
            w354 = 0 ("Top Row")
            n217 = property on="Listbox" class="LstBox (strict)"() -> ("Number of Rows"=w356:u32)  [unwired: 2 in, 2 out]
            n218 = Initialize Array(0, w356) -> (w355:i32[])
            n219 = property on="Listbox" class="LstBox (strict)"("Top Row"=w354, "Value"=w354, "Item Symbols"=w355) -> ()  [unwired: 2 in, 2 out]
          }
        }
      }
      event "Listbox": Key Down {
        # "Update symbols on the listbox\nLeft and right keys check and uncheck"
        n220 = event-data() -> ("VKey"=w360:T32)  [unwired: 1 in]
        n221 = case shown="\"Left\", \"Right\"" w360 {
          selector: w360 -> [w365 _]
          tunnel: eventvkey."Left" ("VKey") -> [w363 _]
          frame "Left", "Right" {
            n222 = Equal?(x=w363, y=w365) -> (x = y?=w364:bool)
            n223 = Select(t=0, s=w364, f=1) -> (s? t:f=w366:i32)
            n224 = property on="Listbox" class="LstBox (strict)"() -> ("Item Symbols"=w369:i32[])  [unwired: 2 in, 2 out]
            n225 = Replace Array Subset(array=w369, new element=w366, index="Listbox") -> (w368:i32[])
            n226 = property on="Listbox" class="LstBox (strict)"("Item Symbols"=w368) -> ()  [unwired: 2 in, 2 out]
          }
          frame Default {
          }
        }
      }
      event "DB Camera Config": Value Change {
        # "Show or hide the cluster of controls, store in ini file"
        n227 = event-data() -> ("NewVal"=w373:bool)  [unwired: 1 in]
        n228 = case shown="False" w373 {
          tunnel: w372 -> [w382 _]
          tunnel: [w375 w393] -> w371
          tunnel: w370 -> [w374 w393]
          frame False {
            w389 = "Camera"
            w392 = FALSE ("Visible")
            n229 = local read "Camera Settings"() -> (w381:T7)
            n230 = Index Array(array=w382) -> (element=w385:cluster{string[]})  [unwired: 1 in]
            n231 = Unbundle(w381) -> ("Frame Rate"=w380:i32, "Compression"=w379:i32, "Size"=w383:u16)
            n232 = Unbundle(w385) -> (w384:string[])
            n233 = Index Array(array=w384, index=w383) -> (element=w378:string)
            n234 = call-poly <vilib>:"Write Key.vi"("section"=w389, "value"=w378, "key"="Size", "refnum"=w374) -> ("refnum out"=w391:T30)  [unwired: 2 in, 5 out]
            n235 = call-poly <vilib>:"Write Key.vi"("section"=w389, "value"=w380, "key"="FrameRate", "refnum"=w391) -> ("refnum out"=w390:T30)  [unwired: 1 in, 6 out]
            n236 = property on="Camera Settings" class="Clust (strict)"("Visible"=w392) -> ()  [unwired: 2 in, 2 out]
            n237 = local write "DB Camera Config"(w392) -> ()
            n238 = call-poly <vilib>:"Write Key.vi"("section"=w389, "value"=w379, "key"="Compression", "refnum"=w390) -> ("refnum out"=w376:T30)  [unwired: 1 in, 6 out]
            n239 = call <vilib>:"Close Config Data.vi"("refnum"=w376) -> ("file path"=w377:path)  [unwired: 2 in, 8 out]
            n240 = call <vilib>:"Open Config Data.vi"("configuration file path"=w377) -> ("refnum"=w375:T30)  [unwired: 8 in, 2 out]
          }
          frame True {
            n241 = property on="Camera Settings" class="Clust (strict)"("Visible"=TRUE) -> ()  [unwired: 2 in, 2 out]
          }
        }
      }
      event "Camera Settings": Value Change {
        # "Update summary string when any elements of DB camera change"
        n242 = event-data() -> ("NewVal"=w406:T7)  [unwired: 1 in]
        n243 = Index Array(array=w402) -> (element=w401:cluster{string[]})  [unwired: 1 in]
        n244 = Unbundle(w406) -> ("Frame Rate"=w397:i32, "Compression"=w396:i32, "Size"=w399:u16)
        n245 = Unbundle(w401) -> (w400:string[])
        n246 = Index Array(array=w400, index=w399) -> (element=w398:string)
        n247 = Format Into String(format string="%s   %dfps   %d%%", w398, w397, w396) -> (resulting string=w403:string)  [unwired: 2 in, 1 out]
        n248 = Build Array(w403) -> (w404:string[])
        n249 = property on="DB Camera Config" class="Bool (strict)"("Strings [4]"=w404) -> ()  [unwired: 2 in, 2 out]
      }
      event "Motor.Enable": Value Change {
        # "When the test mode otor enable helper is set, update that\ntree row item's value"
        n250 = event-data() -> ("NewVal"=w412:bool)  [unwired: 1 in]
        n251 = Unbundle("Motor") -> ("Value"=w411:dbl)  [unwired: 1 out]
        n252 = Select(t=w411, s=w412, f=0.0) -> (s? t:f=w409:dbl)
        n253 = call <vilib>:"NT Write Number.vi"("Numeric"=w409, "Name"=w408) -> ()  [unwired: 9 in, 1 out]
      }
      event "Test Slider": Value Change {
        # "When the test mode slider helper is set, update that\ntree row item's value"
        n254 = event-data() -> ("NewVal"=w415:dbl)  [unwired: 1 in]
        n255 = call <vilib>:"NT Write Number.vi"("Numeric"=w415, "Name"=w416) -> ()  [unwired: 9 in, 1 out]
      }
      event "On/Off": Value Change {
        # "When the test mode on/off helper value is set, update that\ntree row item's value"
        n256 = event-data() -> ("NewVal"=w420:bool)  [unwired: 1 in]
        n257 = Boolean To (0,1)(Boolean=w420) -> (0, 1=w419:i16)
        n258 = call <vilib>:"NT Write Number.vi"("Numeric"=w419, "Name"=w418) -> ()  [unwired: 9 in, 1 out]
      }
      event "Rev/Fwd": Value Change {
        # "When the test mode helper value for relays is set, update that\ntree row item's value"
        n259 = event-data() -> ("NewVal.Forward"=w428:bool, "NewVal.Reverse"=w427:bool)  [unwired: 1 in]
        n260 = Boolean To (0,1)(Boolean=w428) -> (0, 1=w424:i16)
        n261 = Boolean To (0,1)(Boolean=w427) -> (0, 1=w426:i16)
        n262 = Negate(x=w426) -> (-x=w425:i16)
        n263 = Add(x=w424, y=w425) -> (x+y=w423:i16)
        n264 = call <vilib>:"NT Write Number.vi"("Numeric"=w423, "Name"=w422) -> ()  [unwired: 9 in, 1 out]
      }
      event "Test Ring": Value Change {
        # "When a test mode helper value is selected from the ring,\nset the tree item's variable to the string value"
        n265 = event-data() -> ("NewVal"=w432:u16)  [unwired: 1 in]
        n266 = property on="Test Ring" class="Ring (strict)"() -> ("Strings []"=w433:string[])  [unwired: 2 in, 2 out]
        n267 = Index Array(array=w433, index=w432) -> (element=w431:string)
        n268 = call <vilib>:"NT Write String.vi"("String"=w431, "Name"=w430) -> ()  [unwired: 9 in, 1 out]
      }
      event "Rec Mode": Value Change {
        # "Update globals for recording mode and path to read log from.\nClear when logging and let NetworkTables set path for vision to\nuse."
        n269 = event-data() -> ("NewVal"=w443:enum32{"Stop", "Record", "Playback"})  [unwired: 1 in]
        n270 = global write "WPI_DashboardLogging Global.vi" "Logging Filename"(path "") -> ()
        n271 = case shown="\"Playback\"" w443 {
          tunnel: w442 -> [_ w445 w453]
          tunnel: [_ _ w452] -> w439
          tunnel: [_ _ w451] -> _
          tunnel: w437 -> [_ _ w449]
          tunnel: cluster{i32, i32} {-250, 170} -> [_ _ w448]
          tunnel: [_ _ T33 {"Image Size"=TRUE, "Image Type"=TRUE, "Pixel Value"=TRUE, "ROI Information"=TRUE, "Zoom Factor"=FALSE} ("Image Information Shown:All Elements")] -> w435
          tunnel: [_ _ TRUE ("Zoom Factor")] -> w434
          frame Default {
          }
          frame "Stop", "Record" {
            # "Place Window too"
            n272 = invoke class="VI" method="FP.Close"(reference=w445) -> (reference out=w444:refnum<vi>)  [unwired: 2 in, 2 out]
            n273 = invoke class="VI" method="Abort VI"(reference=w444) -> ()  [unwired: 2 in, 3 out]
          }
          frame "Playback" {
            n274 = call "Open Playback Panel.vi"("Offset"=w448, "DB VI Ref"=w449, "Playback in"=w453) -> ("Playback out"=w450:refnum<vi>)  [unwired: 8 in]
            n275 = register-events(w450) -> (reference out=w452:refnum<event-registration>, error out=w451:errorcluster)  [unwired: 2 in]
          }
        }
        n276 = global write "WPI_DashboardLogging Global.vi" "Recording"(w443) -> ()
        n277 = property on="Camera Image" class="ImageControl"("Image Information Shown"=w435, "Image Information Visible"=w434) -> ()  [unwired: 2 in, 2 out]
        n278 = call <vilib>:"WPI_DashboardNT Log FieldName Cache.vi"("Operation"=enum16{"Lookup/Add", "Index", "Clear"}."Clear") -> ()  [unwired: 8 in, 3 out]
      }
      event Panel Close {
        w454 = enum32{"Stop", "Record", "Playback"}."Stop" ("Rec Mode")
        # "Playback window has been closed, abort"
        n279 = event-data() -> ()  [unwired: 1 in, 4 out]
        n280 = local write "Rec Mode"(w454) -> ()
        n281 = global write "WPI_DashboardLogging Global.vi" "Recording"(w454) -> ()
      }
      event Panel Close {
        # "Abort playback window and ourself"
        n282 = event-data() -> ()  [unwired: 1 in, 4 out]
        n283 = invoke class="VI" method="FP.Close"(reference=w459) -> (reference out=w458:refnum<vi>)  [unwired: 2 in, 2 out]
        n284 = invoke class="VI" method="Abort VI"(reference=w458) -> (error out=w457:errorcluster)  [unwired: 2 in, 2 out]
        n285 = invoke class="VI" method="Abort VI"(error in=w457) -> ()  [unwired: 2 in, 3 out]
      }
      event "Vision": Value Change {
        # "Enable/Disable Compression slider.\nHW USB is hard-coded into the camera"
        n286 = event-data() -> ("NewVal"=w465:u16)  [unwired: 1 in]
        n287 = Equal?(x=w465, y=u32 2 ("milliseconds to wait")) -> (x = y?=w463:bool)
        n288 = Select(t=T34."Disabled and Grayed Out" ("Disabled"), s=w463, f=T34."Enabled" ("Disabled")) -> (s? t:f=w460:T34)
        n289 = property on="Compression" class="Slide (strict)"("DisabledEnum"=w460) -> ()  [unwired: 2 in, 2 out]
      }
    }
  }
  n290 = while {
    tunnel: w42 -> [w468]
    i -> [w471]
    stop <- FALSE stop-if-true
    n291 = Wait (ms)(milliseconds to wait=u32 100) -> ()  [unwired: 1 out]
    n292 = case shown="\"Playback\"" "Rec Mode" {
      tunnel: w471 -> [_ _ w486]
      tunnel: [u32 2829099 ("Base Color") u32 11141120 ("Target Color") w475] -> w467
      frame "Stop", Default {
        # "Reset the color, extra updates don't cost much"
      }
      frame "Record" {
      }
      frame "Playback" {
        # "Playback"
        n293 = Quotient & Remainder(x=w486, y=u32 50 ("milliseconds to wait")) -> (x-y*floor(x/y)=w482:u32)  [unwired: 1 out]
        n294 = Divide(x=w482, y=u32 50 ("milliseconds to wait")) -> (x/y=w479:dbl)
        n295 = Multiply(x=6.283185307179586, y=w479) -> (x*y=w484:dbl)
        n296 = Sine(x=w484) -> (sin(x)=w483:dbl)
        n297 = Absolute Value(x=w483) -> (abs(x)=w476:dbl)
        n298 = call "Interpolate RGB Color.vi"("Proportion"=w476, "Target Color"=u32 30976, "Base Color"=u32 2829099) -> ("Result Color"=w475:u32)  [unwired: 8 in]
      }
    }
    n299 = property class="Pane"(reference=w468, "PaneColor"=w467) -> ()  [unwired: 1 in, 2 out]
  }
  n300 = TCP Create Listener(10:u16 1741 ("timeout ms (25000)")) -> (3:w5:refnum<k5>)  [unwired: 4 in, 2 out]
  n301 = while {
    tunnel: w5 -> [w488]
    stop <- FALSE stop-if-true
    n302 = TCP Wait On Listener(11:w488) -> (4:w487:refnum<k5>)  [unwired: 3 in, 4 out]
    n303 = local write "TCP"(w487) -> ()
  }
  n304 = property on="On/Off" class="Bool (strict)"("Visible"=w10) -> ()  [unwired: 2 in, 2 out]
  n305 = property on="Motor" class="Clust (strict)"("Visible"=w10) -> ()  [unwired: 2 in, 2 out]
  n306 = property on="Progress" class="Clust (strict)"("Visible"=w10) -> ()  [unwired: 2 in, 2 out]
  n307 = property on="Test Ring" class="Ring (strict)"("Visible"=w10) -> ()  [unwired: 2 in, 2 out]
  n308 = property on="Rev/Fwd" class="Clust (strict)"("Visible"=w10) -> ()  [unwired: 2 in, 2 out]
  n309 = property on="Camera Settings" class="Clust (strict)"("Visible"=w10) -> ()  [unwired: 2 in, 2 out]
  n310 = local write "DB Camera Config"(w10) -> ()
  n311 = global write "WPI_DashboardLogging Global.vi" "Recording"(w36) -> ()
  n312 = local write "Rec Mode"(w36) -> ()
